vi "KM_peak -- find -- pm - V1.vi"(0 "omega in":dbl[](array[numeric]), 1 "z in":cdb[](array[numeric]), 5 "parameters: complex fit":T4={"main VI path"=path "", "scale factor"=3.0, "# of grid points"=200, "parameters: wavepacket"={"R"=0.5, "wave number"=22.0, "delta k"=7.0, "radii vector"=[], "radial section"=[], "wave vector"=22.0, "wavepacket is"=TRUE}, "span"=0.27789, "interference ?"=enum."cp z center", "filter method"=enum."three"} {"span" min=0.0 max=0.5 step=1e-05 scale=0.0001..0.5 scale format="%#_5f"; "parameters: wavepacket"."delta k" format="%#_3f"; "parameters: wavepacket"."wave number" format="%#_3f"; "parameters: wavepacket"."R" format="%#_3f"}, 7 "plots: filter related":T3, 8 "plot staff ?":enum16{"plot", "do not plot", "a"}(ring), 9 "just guess?":bool, 11 "subtract linear BG":bool) -> (17 "good lorentzian":T1={"A (VHz)"=-1.0311345636926572, "f (Hz)"=-1.0311345636926572, "G (Hz)"=-1.0311345636926572, "phi(rad)"=-1.0311345636926572, "Q"=-1.0311345636926572, "Norm  Ampl"=-1.0311345636926572, "bg (V)"=-1.0311345636926572+0.0i, "4corners"={"z (-pi/2)"=-1.0311345636926572+0.5736824521422934i, "z(inf)"=-0.5200164984937075+1.0975277942502903i, "z (pi/2)"=-1.0311345636926572+0.5736824521422934i, "z center"=-0.5136528600391839+0.580046090596817i, "z(0)"=-0.5200164984937075+1.0975277942502903i, "radius"=-1.0311345636926572}} {"bg (V)" format="%#9_9f"; "Q" format="%#9_9f"; "phi(rad)" format="%#9_9f"; "G (Hz)" format="%#9_9f"; "f (Hz)" format="%#9_9f"}, 18 "pm lorentzian":T1={"A (VHz)"=-1.0311345636926572, "f (Hz)"=-1.0311345636926572, "G (Hz)"=-1.0311345636926572, "phi(rad)"=-1.0311345636926572, "Q"=-1.0311345636926572, "Norm  Ampl"=-1.0311345636926572, "bg (V)"=-1.0311345636926572+0.0i, "4corners"={"z (-pi/2)"=-1.0311345636926572+0.5736824521422934i, "z(inf)"=-0.5200164984937075+1.0975277942502903i, "z (pi/2)"=-1.0311345636926572+0.5736824521422934i, "z center"=-0.5136528600391839+0.580046090596817i, "z(0)"=-0.5200164984937075+1.0975277942502903i, "radius"=-1.0311345636926572}} {"bg (V)" format="%#9_9f"; "Q" format="%#9_9f"; "phi(rad)" format="%#9_9f"; "G (Hz)" format="%#9_9f"; "f (Hz)" format="%#9_9f"}, 19 "cp lorentzian":T1={"A (VHz)"=-1.0311345636926572, "f (Hz)"=-1.0311345636926572, "G (Hz)"=-1.0311345636926572, "phi(rad)"=-1.0311345636926572, "Q"=-1.0311345636926572, "Norm  Ampl"=-1.0311345636926572, "bg (V)"=-1.0311345636926572+0.0i, "4corners"={"z (-pi/2)"=-1.0311345636926572+0.5736824521422934i, "z(inf)"=-0.5200164984937075+1.0975277942502903i, "z (pi/2)"=-1.0311345636926572+0.5736824521422934i, "z center"=-0.5136528600391839+0.580046090596817i, "z(0)"=-0.5200164984937075+1.0975277942502903i, "radius"=-1.0311345636926572}} {"bg (V)" format="%#9_9f"; "Q" format="%#9_9f"; "phi(rad)" format="%#9_9f"; "G (Hz)" format="%#9_9f"; "f (Hz)" format="%#9_9f"})   [LabVIEW 2018]
uses:
  filter method control.ctl
  circle corners.ctl
  lorentzian.ctl
  wavepacket.ctl
  peak -- parameters -- complex fit.ctl
  plot refs -- filter related.ctl
panel:
  in  "span":dbl=0.01
  in  "filter method":T6=enum."three"
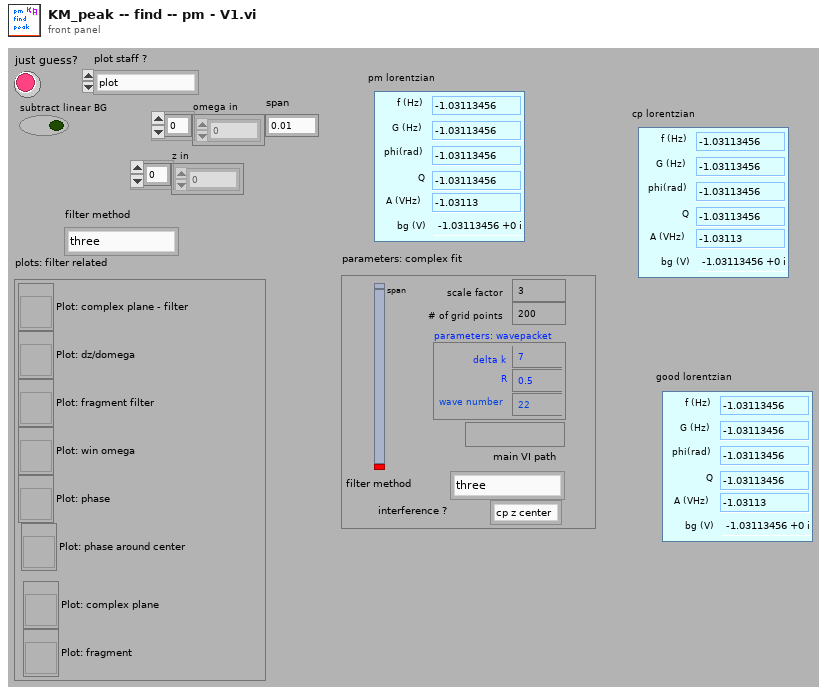
[diagram p1: front panel]
types:
  T1 = typedef "lorentzian.ctl" = cluster{"A (VHz)":dbl, "f (Hz)":dbl, "G (Hz)":dbl, "phi(rad)":dbl, "Q":dbl, "Norm  Ampl":dbl, "bg (V)":cdb, "4corners":T2}
  T2 = typedef "circle corners.ctl" = cluster{"z (-pi/2)":cdb, "z(inf)":cdb, "z (pi/2)":cdb, "z center":cdb, "z(0)":cdb, "radius":dbl}
  T3 = typedef "plot refs -- filter related.ctl" = cluster{"Plot: complex plane - filter":refnum<vi>, "Plot: dz/domega":refnum<vi>, "Plot: fragment filter":refnum<vi>, "Plot: win omega":refnum<vi>, "Plot: phase":refnum<vi>, "Plot: phase around center":refnum<vi>, "Plot: complex plane":refnum<vi>, "Plot: fragment":refnum<vi>}
  T4 = typedef "peak -- parameters -- complex fit.ctl" = cluster{"main VI path":path, "scale factor":dbl, "# of grid points":i32, "parameters: wavepacket":T5, "span":dbl, "interference ?":enum16{"cp z center", "pm zcenter", "fancy"}, "filter method":T6}
  T5 = typedef "wavepacket.ctl" = cluster{"R":dbl, "wave number":dbl, "delta k":dbl, "radii vector":dbl[], "radial section":cdb[], "wave vector":dbl, "wavepacket is":bool}
  T6 = typedef "filter method control.ctl" = enum16{"four", "five", "one", "two", "three", "zero", "minus one", "minus two"}
  T7 = typedef "tale of three indices -- int -- control.ctl" = cluster{"left":i32, "center":i32, "right":i32, "right most":i32, "left most":i32, "window":i32, "max win factor":i32, "max win":i32, "min win":i32}
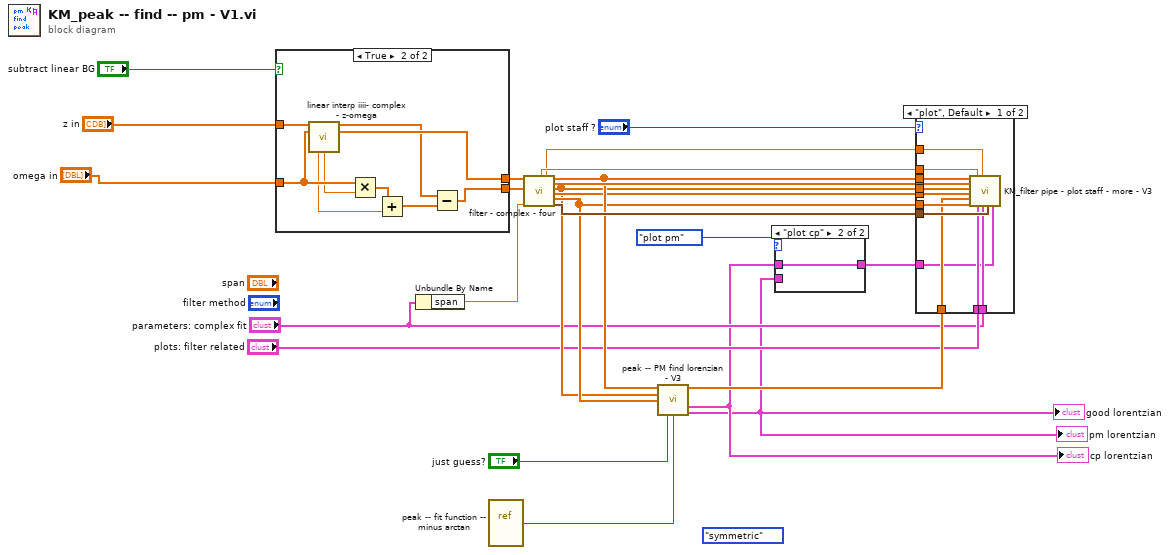
[diagram p0: block diagram]
diagram:
  (unwired) enum16{"symmetric", "skewed", "fancy"}."symmetric" ("kind")
  n1 = case shown="True" "subtract linear BG" {
    tunnel: "omega in" -> [w26 w33]
    tunnel: "z in" -> [w25 w35]
    tunnel: [w25 w27] -> w7
    tunnel: [w26 w34] -> w6
    frame False {
    }
    frame True {
      n2 = call "linear interp iiii- complex - z-omega.vi"("z"=w35, "omega"=w33) -> ("z out"=w29:cdb[], "omega out"=w34:dbl[], "intercept"=w30:cdb, "slope"=w32:cdb)  [unwired: 5 in, 5 out]
      n3 = Multiply(x=w33, y=w32) -> (x*y=w31:cdb[])
      n4 = Add(x=w31, y=w30) -> (x+y=w28:cdb[])
      n5 = Subtract(x=w29, y=w28) -> (x-y=w27:cdb[])
    }
  }
  n6 = Unbundle By Name("parameters: complex fit") -> ("span"=w13:dbl)
  n7 = vi-ref "peak -- fit function -- minus arctan.vi"() -> (w1:refnum<vi>)
  n8 = call "filter - complex - four.vi"("omega  in"=w6, "z in"=w7, "span"=w13) -> ("center"=w21:cdb, "norm"=w20:dbl, "omega out"=w22:dbl[], "z in out"=w23:cdb[], "z out"=w16:cdb[], "win omega out"=w19:dbl[], "dz/domega out"=w18:cdb[], "tale of three"=w24:T7)  [unwired: 9 in]
  n9 = call "peak -- PM find lorenzian - V3.vi"("omega"=w22, "z"=w16, "dz/domega"=w18, "just guess?"="just guess?", "VI Refnum"=w1) -> ("phase (around center)"=w17:dbl[], "cp lorentzian"=w11:T1, "poor man lorentzian"=w10:T1)  [unwired: 7 in, 1 out]
  "pm lorentzian" <- w10
  "cp lorentzian" <- w11
  "good lorentzian" <- w10
  n10 = case shown="\"plot cp\"" enum16{"plot pm", "plot cp", "a"}."plot pm" ("plot what") {
    tunnel: [w36 w37] -> w3
    tunnel: w11 -> [_ w37]
    tunnel: w10 -> [w36 _]
    frame "plot pm", Default {
    }
    frame "plot cp" {
    }
  }
  n11 = case shown="\"plot\", Default" "plot staff ?" {
    tunnel: w24 -> [w49 _]
    tunnel: w23 -> [w48 _]
    tunnel: w22 -> [w47 _]
    tunnel: w21 -> [w46 _]
    tunnel: w20 -> [w45 _]
    tunnel: w19 -> [w44 _]
    tunnel: w18 -> [w43 _]
    tunnel: w17 -> [w42 _]
    tunnel: w16 -> [w41 _]
    tunnel: "plots: filter related" -> [w40 _]
    tunnel: "parameters: complex fit" -> [w39 _]
    tunnel: w3 -> [w38 _]
    frame "plot", Default {
      n12 = call "KM_filter pipe - plot staff - more - V3.vi"("omega  in"=w47, "zin"=w48, "z out"=w41, "win omega"=w44, "phase"=w42, "dz/domega in"=w43, "center"=w46, "plots: filter related"=w40, "norm"=w45, "parameters: complex fit"=w39, "tale of three indices -- int -- control"=w49, "lorentzian"=w38) -> ()  [unwired: 8 in]
    }
    frame "do not plot" {
    }
  }
